vi "GOOP_AddCustomClassTemplates.vi"(1 "TemplateIdNames":T1[](array[typedef]), 2 "String":string) -> (0 "TemplateIdNames 2":T1[](array[typedef]))   [LabVIEW 2020]
uses:
  <resource>/Framework/Providers/Open_GDS/ClassProviders/Provider_BaseClassInterface/ClassTemplateType.ctl
  <resource>/Framework/Providers/Open_GDS/ClassProviders/Provider_BaseClassInterface/ClassWriter_class/ClassWriter.lvclass
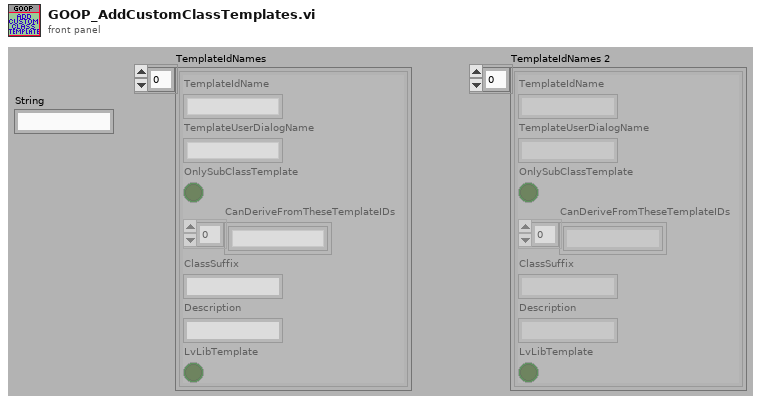
[diagram p1: front panel]
types:
  T1 = typedef "ClassWriter.lvclass/ClassTemplateType.ctl" = cluster{"TemplateIdName":string, "TemplateUserDialogName":string, "OnlySubClassTemplate":bool, "CanDeriveFromTheseTemplateIDs":string[], "ClassSuffix":string, "Description":string, "LvLibTemplate":bool}
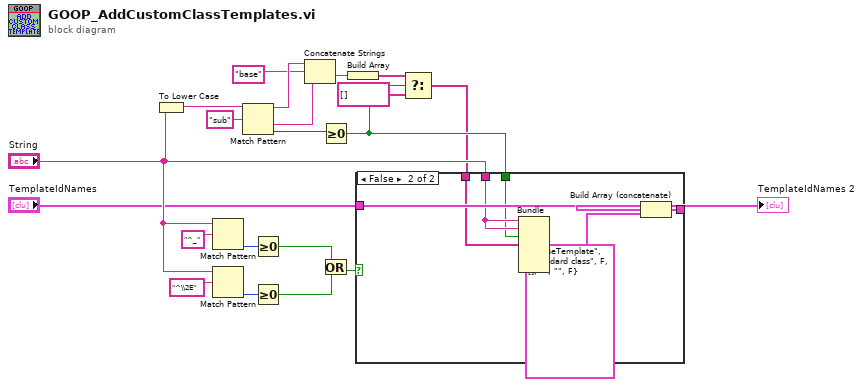
[diagram p0: block diagram]
diagram:
  n1 = To Lower Case(string="String") -> (all lower case string=w19:string)
  n2 = Match Pattern(string="String", regular expression="^_") -> (offset past match=w11:i32)  [unwired: 1 in, 3 out]
  n3 = Match Pattern(string="String", regular expression="^\\2E") -> (offset past match=w14:i32)  [unwired: 1 in, 3 out]
  n4 = Match Pattern(string=w19, regular expression="sub") -> (before substring=w8:string, after substring=w7:string, offset past match=w20:i32)  [unwired: 1 in, 1 out]
  n5 = Greater Or Equal To 0?(x=w11) -> (x >= 0?=w15:bool)
  n6 = Greater Or Equal To 0?(x=w14) -> (x >= 0?=w16:bool)
  n7 = Concatenate Strings(w8, "base" ("regular expression"), w7) -> (w4:string)
  n8 = Greater Or Equal To 0?(x=w20) -> (x >= 0?=w5:bool)
  n9 = Or(x=w15, y=w16) -> (x .or. y?=w17:bool)
  n10 = Build Array(w4) -> (w3:string[])
  n11 = Select(t=w3, s=w5, f=string[] []) -> (s? t:f=w2:string[])
  n12 = case shown="False" w17 {
    tunnel: [w22 w29] -> w9
    tunnel: "TemplateIdNames" -> [w22 w28]
    tunnel: "String" -> [_ w25]
    tunnel: w5 -> [_ w24]
    tunnel: w2 -> [_ w23]
    frame True {
    }
    frame False {
      n13 = Bundle(cluster=T1 {"TemplateIdName"="BaseTemplate", "TemplateUserDialogName"="Standard class", "OnlySubClassTemplate"=FALSE, "CanDeriveFromTheseTemplateIDs"=[], "ClassSuffix"="", "Description"="", "LvLibTemplate"=FALSE} ("ClassTemplateType"), "TemplateIdName"=w25, "TemplateUserDialogName"=w25, "OnlySubClassTemplate"=w24, "CanDeriveFromTheseTemplateIDs"=w23) -> (w26:T1)  [unwired: 3 in]
      n14 = Build Array (concatenate)(w28, w26) -> (w29:T1[])
    }
  }
  "TemplateIdNames 2" <- w9
